vi "HVAC Randomize Statuses.vi"(10 "DeviceID":T2) -> (3 "HVAC_Status Array out":T1[](array[typedef]))   [LabVIEW 2018, in "IED Test Framework.lvlib" / "IED Test.lvclass"]
uses:
  IED Test.lvclass
  <vilib>/ORNL/CSEISMIC DDS/CSEISMIC DDS Base/Data Types/Controls/DeviceID.ctl
  <vilib>/ORNL/CSEISMIC DDS/CSEISMIC DDS Base/Data Types/HVAC_Status.ctl
  <vilib>/ORNL/CSEISMIC DDS/CSEISMIC DDS Base/Data Types/Controls/ControlMode.ctl
  <vilib>/ORNL/CSEISMIC DDS/CSEISMIC DDS Base/CSEISMIC DDS.lvclass
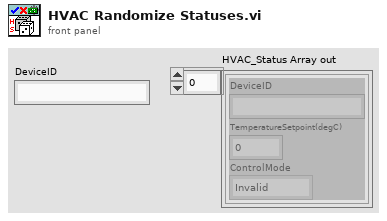
[diagram p1: front panel]
types:
  T1 = typedef "CSEISMIC DDS.lvlib/CSEISMIC DDS.lvclass/HVAC_Status.ctl" = cluster{"DeviceID":T2, "TemperatureSetpoint(degC)":dbl, "ControlMode":T3}
  T2 = typedef "CSEISMIC DDS.lvlib/CSEISMIC DDS.lvclass/DeviceID.ctl" = string
  T3 = typedef "CSEISMIC DDS.lvlib/CSEISMIC DDS.lvclass/ControlMode.ctl" = enum32{"Invalid", "Cooling", "Heating"}
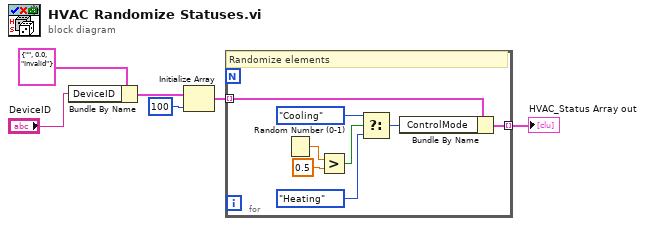
[diagram p0: block diagram]
diagram:
  n1 = Bundle By Name(cluster=T1 {"DeviceID"="", "TemperatureSetpoint(degC)"=0.0, "ControlMode"=enum."Invalid"} ("HVAC_Status"), "DeviceID"="DeviceID") -> (w6:T1)
  n2 = Initialize Array(w6, 100 ("dimension size")) -> (w3:T1[])
  n3 = for {
    tunnel: w3 -> [w14] mode=indexing
    tunnel: [w13] -> w2 mode=indexing
    # "Randomize elements"
    n4 = Random Number (0-1)() -> (number: 0 to 1=w12:dbl)
    n5 = Greater?(x=w12, y=0.5) -> (0:w10:bool)
    n6 = Select(t=ControlMode."Cooling" ("ControlMode"), s=w10, f=ControlMode."Heating" ("ControlMode")) -> (s? t:f=w7:T3)
    n7 = Bundle By Name(cluster=w14, "ControlMode"=w7) -> (w13:T1)
  }
  "HVAC_Status Array out" <- w2
